vi "Change Host Time.vi"(8 "error in":errorcluster, 11 "tCRD in":refnum<class "Aircraft OPCCRD.lvclass">) -> (0 "error out":errorcluster, 3 "tCRD out":refnum<class "Aircraft OPCCRD.lvclass">)   [LabVIEW 2015, in "Aircraft OPCCRD.lvclass"]
doc: "Set the time on the board."
uses:
  Aircraft OPCCRD.lvclass
  <vilib>/nisyscfg/nisyscfg.lvlib
  Reusable/Instrument/Instrument.lvclass
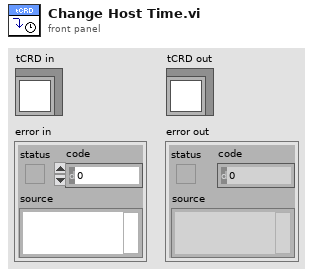
[diagram p1: front panel]
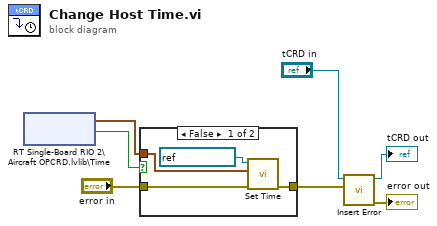
[diagram p0: block diagram]
diagram:
  n1 = shared-variable "RT Single-Board RIO 2\\Aircraft OPCRD.lvlib\\Time"() -> (w6:timestamp, w7:bool)  [unwired: 2 in, 1 out]
  n2 = case shown="False" w7 {
    tunnel: w6 -> [w11 _]
    tunnel: "error in" -> [w9 w12]
    tunnel: [w8 w12] -> w4
    frame False {
      n3 = call <vilib>:"Set Time.vi"("error in (no error)"=w9, "Time"=w11, "Session in (localhost)"=refnum<k21> "localhost" ("session in (localhost)")) -> ("error out"=w8:errorcluster)  [unwired: 5 in, 3 out]
    }
    frame True {
    }
  }
  n4 = call "Insert Error.vi"("err"=w4, "Instrument in"="tCRD in") -> ("error out"=→"error out":errorcluster, "Instrument out"=→"tCRD out":refnum<class "Aircraft OPCCRD.lvclass">)  [unwired: 7 in, 1 out]
